vi "motion_generate_test_withvelocitycontrol_withswingdelay_motor4.vi"() -> ()   [LabVIEW 2017]
uses:
  Downloads/Interfacing File 1/Software_Driver/DynamixelSDK/DynamixelSDK-master/labview/dxl_x86_c.lvlib/dxl_x86_c.lvlib
panel:
  in  "ADDR_MX_GOAL_Velocity 2":u8=5
  in  "data 3":u16
  in  "data 2":u16
  in  "data":u16
  in  "ADDR_MX_GOAL_Velocity":u8=5
  in  "angle 2":dbl=180.0
  in  "motor3 2":dbl=220.0
  in  "motor1&2 2":dbl=150.0
  in  "z축 선택":dbl
  in  "motor1&2":dbl=150.0
  in  "motor3":dbl=220.0
  in  "angle":dbl=180.0
  in  "Boolean":bool
  in  "positioning time_2":u32
  in  "positioning time_1":u32
  in  "initial_5":dbl=230.0
  in  "initial_4":dbl=180.0
  out "value : MX (knob)\npresent position 4":u16(knob)
  in  "dynamixel_id 4":u8=4
  out "protocol_version 2":dbl=2.0
  in  "ADDR_MX_\nPRESENT_POSITION 2":u16=132
  out "dynamixel_error 2":string
  out "dynamixel_comm_result  2":string
  in  "ADDR_MX_\nGOAL_POSITION 2":u16=116
  in  "ADDR_MX_\nTORQUE_ENABLE 2":u16=64
  in  "initial_3":dbl=260.0
  in  "initial_1&2":dbl=230.0
  out "value : MX (knob)\npresent position 3":u16(knob)
  out "value : MX (knob)\npresent position 2":u16(knob)
  out "value : MX (knob)\npresent position":u16(knob)
  in  "dynamixel_id 3":u8=3
  in  "dynamixel_id 2":u8=2
  out "dynamixel_comm_result":string
  out "dynamixel_error":string
  in  "device_name":string="COM3"
  in  "ADDR_MX_\nPRESENT_POSITION":u16=36
  in  "ADDR_MX_\nGOAL_POSITION":u16=30
  in  "ADDR_MX_\nTORQUE_ENABLE":u16=24
  out "protocol_version":dbl=1.0
  in  "terminate":bool
  out "port_num":i32
  in  "dynamixel_id":u8=1
  in  "baud_rate":i32=57600
  # "Motor connection status"
  # "Time set"
  # "Sensing data"
  # "Handler setup"
  # "link length"
  # "initial angle"
  # "desired angle"
  # "*각 관절에 모터 연결 시 180도 라인 기준으로 연결 시키기 \n(-각도 반영해주기 위함!) \n-> 모터 input은 -180~180까지 계산됨!"
  # "*yaw motor는 0도 라인 기준으로 연결 시키기"
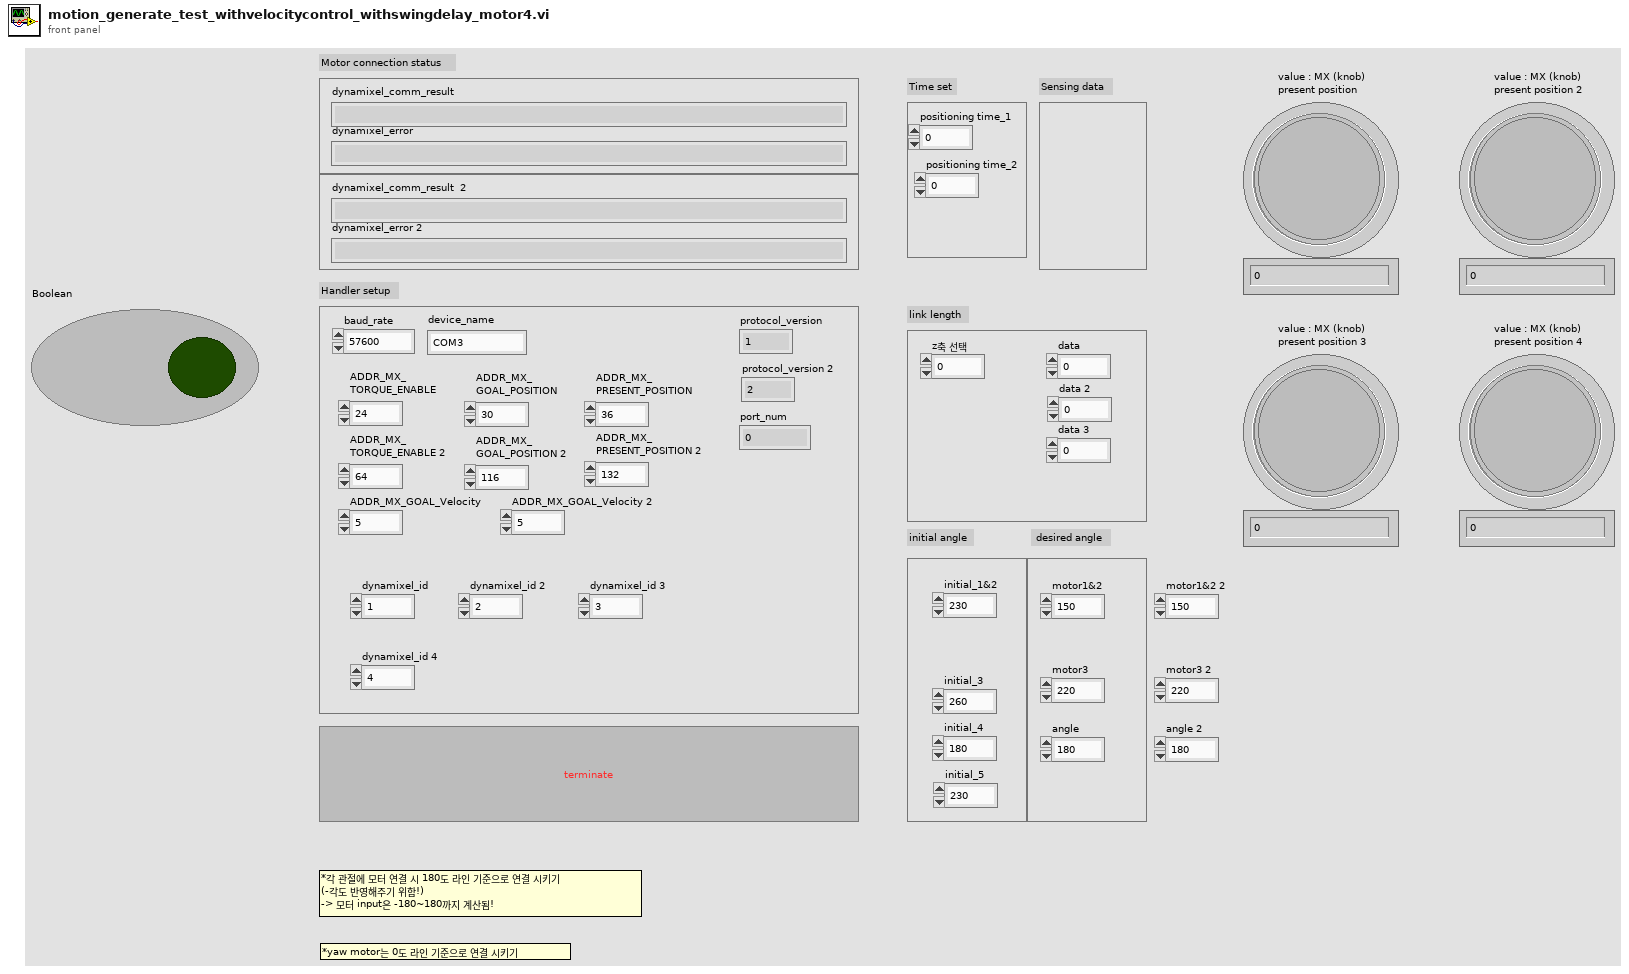
[diagram p1: front panel]
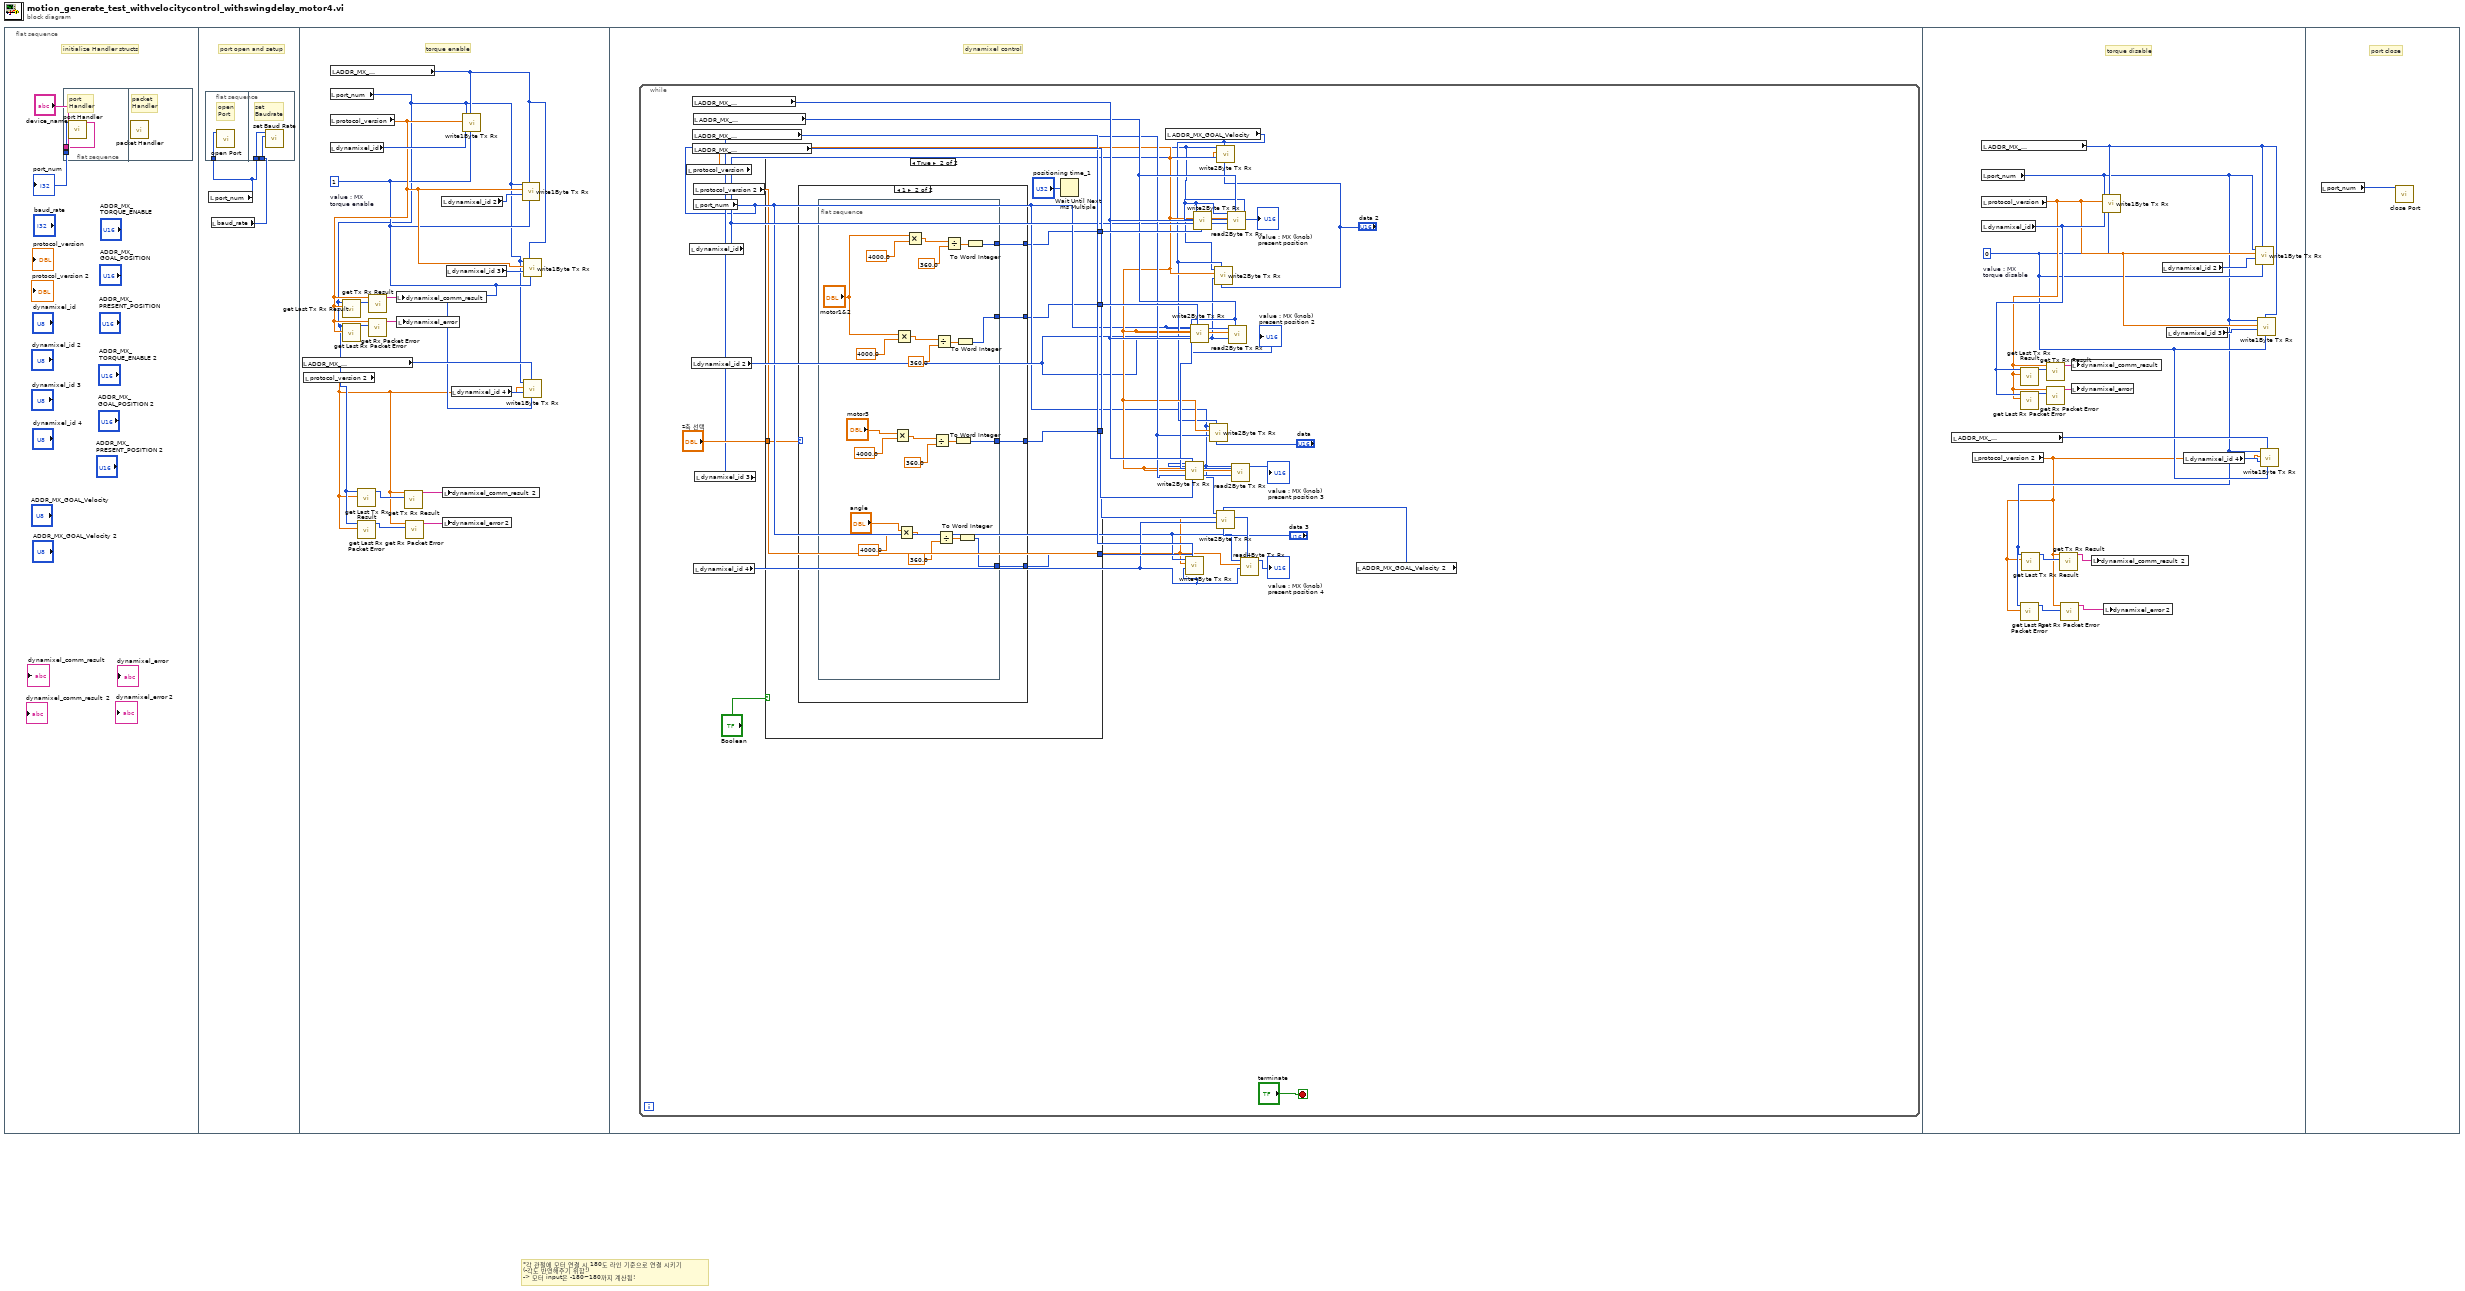
[diagram p0: block diagram]
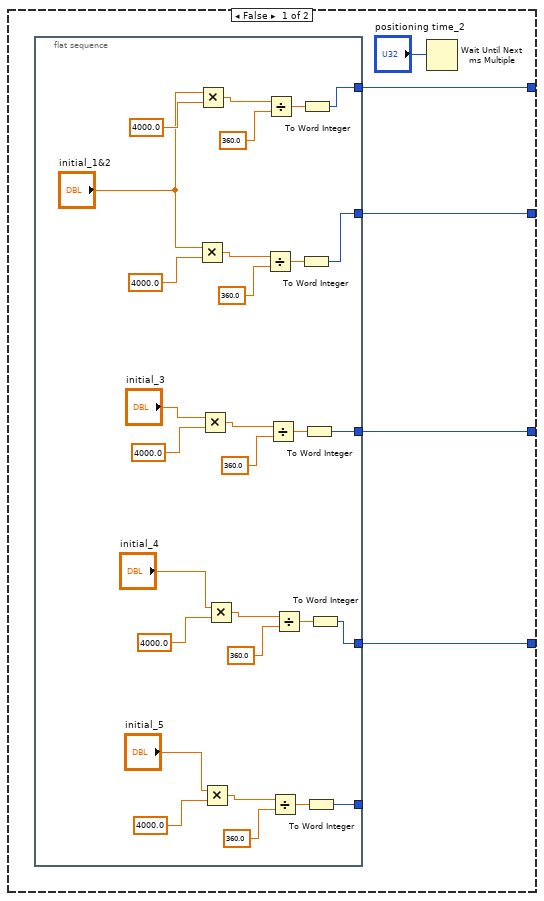
[diagram p2: hidden frame]
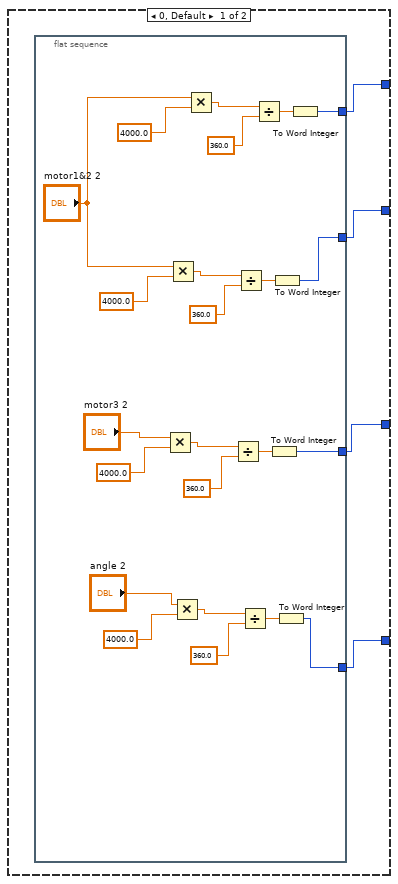
[diagram p3: hidden frame]
diagram:
  # "*각 관절에 모터 연결 시 180도 라인 기준으로 연결 시키기 \n(-각도 반영해주기 위함!) \n-> 모터 input은 -180~180까지 계산됨!"
  n1 = flat-sequence {
    frame #0 {
      # "initialize Handler structs"
      n2 = flat-sequence {
        tunnel: [w4] -> w2
        tunnel: "device_name" -> [w3]
        frame #0 {
          # "port\nHandler"
          n3 = call "port Handler.vi"("port_name"=w3) -> ("function return"=w4:i32)  [unwired: 10 in]
        }
        frame #1 {
          # "packet\nHandler"
          n4 = call "packet Handler.vi"() -> ()  [unwired: 12 in]
        }
      }
      "port_num" <- w2
    }
    frame #1 {
      # "port open and setup"
      n5 = flat-sequence {
        tunnel: w6 -> [w7]
        tunnel: w6 -> [w9]
        tunnel: w5 -> [w8]
        frame #0 {
          # "open\nPort"
          n6 = call "open Port.vi"("port_num"=w7) -> ()  [unwired: 10 in, 1 out]
        }
        frame #1 {
          # "set\nBaudrate"
          n7 = call "set Baud Rate.vi"("baudrate"=w8, "port_num"=w9) -> ()  [unwired: 9 in, 1 out]
        }
      }
      n8 = local read "port_num"() -> (w6:i32)
      n9 = local read "baud_rate"() -> (w5:i32)
    }
    frame #2 {
      w16 = 1  # value : MX torque enable
      # "torque enable"
      n10 = local read "ADDR_MX_\nTORQUE_ENABLE 2"() -> (w17:u16)
      n11 = local read "protocol_version 2"() -> (w10:dbl)
      n12 = local read "port_num"() -> (w11:i32)
      n13 = local read "protocol_version"() -> (w20:dbl)
      n14 = local read "dynamixel_id"() -> (w27:u8)
      n15 = local read "ADDR_MX_\nTORQUE_ENABLE"() -> (w19:u16)
      n16 = call "get Last Tx Rx Result.vi"("protocol_version"=w20, "port_num"=w11) -> ("function return"=w23:i32)  [unwired: 9 in]
      n17 = call "get Last Rx Packet Error.vi"("protocol_version"=w20, "port_num"=w11) -> ("function return"=w24:u8)  [unwired: 9 in]
      n18 = call "get Last Rx Packet Error.vi"("protocol_version"=w10, "port_num"=w11) -> ("function return"=w13:u8)  [unwired: 9 in]
      n19 = call "get Last Tx Rx Result.vi"("protocol_version"=w10, "port_num"=w11) -> ("function return"=w15:i32)  [unwired: 9 in]
      n20 = call "get Rx Packet Error.vi"("error"=w24, "protocol_version"=w20) -> ("function return"=w26:string)  [unwired: 9 in]
      n21 = call "get Tx Rx Result.vi"("result"=w23, "protocol_version"=w20) -> ("function return"=w25:string)  [unwired: 9 in]
      n22 = local write "dynamixel_comm_result"(w25) -> ()
      n23 = local write "dynamixel_error"(w26) -> ()
      n24 = call "get Tx Rx Result.vi"("result"=w15, "protocol_version"=w10) -> ("function return"=w14:string)  [unwired: 9 in]
      n25 = call "get Rx Packet Error.vi"("error"=w13, "protocol_version"=w10) -> ("function return"=w12:string)  [unwired: 9 in]
      n26 = local read "dynamixel_id 2"() -> (w22:u8)
      n27 = local write "dynamixel_comm_result  2"(w14) -> ()
      n28 = local write "dynamixel_error 2"(w12) -> ()
      n29 = local read "dynamixel_id 3"() -> (w21:u8)
      n30 = local read "dynamixel_id 4"() -> (w18:u8)
      n31 = call "write1Byte Tx Rx.vi"("data"=w16, "address"=w19, "id"=w27, "protocol_version"=w20, "port_num"=w11) -> ()  [unwired: 7 in]
      n32 = call "write1Byte Tx Rx.vi"("data"=w16, "address"=w19, "id"=w22, "protocol_version"=w20, "port_num"=w11) -> ()  [unwired: 7 in]
      n33 = call "write1Byte Tx Rx.vi"("data"=w16, "address"=w19, "id"=w21, "protocol_version"=w20, "port_num"=w11) -> ()  [unwired: 7 in]
      n34 = call "write1Byte Tx Rx.vi"("data"=w16, "address"=w17, "id"=w18, "protocol_version"=w10, "port_num"=w11) -> ()  [unwired: 7 in]
    }
    frame #3 {
      # "dynamixel control"
      n35 = while {
        stop <- "terminate" stop-if-true
        n36 = local read "protocol_version"() -> (w36:dbl)
        n37 = local read "dynamixel_id"() -> (w37:u8)
        n38 = local read "dynamixel_id 2"() -> (w35:u8)
        n39 = local read "ADDR_MX_\nGOAL_POSITION"() -> (w51:u16)
        n40 = local read "ADDR_MX_\nGOAL_POSITION 2"() -> (w43:u16)
        n41 = local read "ADDR_MX_\nPRESENT_POSITION 2"() -> (w44:u16)
        n42 = local read "ADDR_MX_\nPRESENT_POSITION"() -> (w50:u16)
        n43 = local read "protocol_version 2"() -> (w29:dbl)
        n44 = local read "port_num"() -> (w30:i32)
        n45 = local read "dynamixel_id 4"() -> (w33:u8)
        n46 = local read "dynamixel_id 3"() -> (w39:u8)
        n47 = case shown="True" "Boolean" {
          tunnel: [w59 w94] -> w53
          tunnel: [w58 w93] -> w52
          tunnel: [w57 w92] -> w49
          tunnel: [w56 w91] -> w42
          tunnel: "z축 선택" -> [_ w89]
          frame False {
            n48 = flat-sequence {
              tunnel: [w84] -> w59
              tunnel: [w74] -> w58
              tunnel: [w73] -> w57
              tunnel: [w64] -> w56
              tunnel: [w63] -> _
              frame #0 {
                n49 = Multiply(x="initial_1&2", y=4000.0) -> (x*y=w82:dbl)
                n50 = Multiply(x="initial_1&2", y=4000.0) -> (x*y=w87:dbl)
                n51 = Multiply(x="initial_3", y=4000.0) -> (x*y=w78:dbl)
                n52 = Multiply(x="initial_5", y=4000.0) -> (x*y=w67:dbl)
                n53 = Multiply(x="initial_4", y=4000.0) -> (x*y=w71:dbl)
                n54 = Divide(x=w82, y=360.0) -> (x/y=w80:dbl)
                n55 = Divide(x=w87, y=360.0) -> (x/y=w85:dbl)
                n56 = Divide(x=w78, y=360.0) -> (x/y=w76:dbl)
                n57 = Divide(x=w67, y=360.0) -> (x/y=w65:dbl)
                n58 = Divide(x=w71, y=360.0) -> (x/y=w69:dbl)
                n59 = To Word Integer(number=w80) -> (16bit integer=w74:i16)
                n60 = To Word Integer(number=w85) -> (16bit integer=w84:i16)
                n61 = To Word Integer(number=w76) -> (16bit integer=w73:i16)
                n62 = To Word Integer(number=w65) -> (16bit integer=w63:i16)
                n63 = To Word Integer(number=w69) -> (16bit integer=w64:i16)
              }
            }
            n64 = Wait Until Next ms Multiple(millisecond multiple="positioning time_2") -> ()  [unwired: 1 out]
          }
          frame True {
            n65 = case shown="1" w89 {
              tunnel: [w95 w125] -> w94
              tunnel: [w96 w124] -> w93
              tunnel: [w97 w123] -> w92
              tunnel: [w98 w122] -> w91
              frame 0, Default {
                n66 = flat-sequence {
                  tunnel: [w117] -> w95
                  tunnel: [w112] -> w96
                  tunnel: [w103] -> w98
                  tunnel: [w99] -> w97
                  frame #0 {
                    n67 = Multiply(x="motor3 2", y=4000.0) -> (x*y=w110:dbl)
                    n68 = Multiply(x="motor1&2 2", y=4000.0) -> (x*y=w115:dbl)
                    n69 = Multiply(x="angle 2", y=4000.0) -> (x*y=w106:dbl)
                    n70 = Multiply(x="motor1&2 2", y=4000.0) -> (x*y=w120:dbl)
                    n71 = Divide(x=w110, y=360.0) -> (x/y=w108:dbl)
                    n72 = Divide(x=w115, y=360.0) -> (x/y=w113:dbl)
                    n73 = Divide(x=w106, y=360.0) -> (x/y=w104:dbl)
                    n74 = Divide(x=w120, y=360.0) -> (x/y=w118:dbl)
                    n75 = To Word Integer(number=w108) -> (16bit integer=w99:i16)
                    n76 = To Word Integer(number=w113) -> (16bit integer=w112:i16)
                    n77 = To Word Integer(number=w104) -> (16bit integer=w103:i16)
                    n78 = To Word Integer(number=w118) -> (16bit integer=w117:i16)
                  }
                }
              }
              frame 1 {
                n79 = flat-sequence {
                  tunnel: [w144] -> w125
                  tunnel: [w139] -> w124
                  tunnel: [w134] -> w123
                  tunnel: [w129] -> w122
                  frame #0 {
                    n80 = Multiply(x="motor3", y=4000.0) -> (x*y=w137:dbl)
                    n81 = Multiply(x="motor1&2", y=4000.0) -> (x*y=w142:dbl)
                    n82 = Multiply(x="angle", y=4000.0) -> (x*y=w132:dbl)
                    n83 = Multiply(x="motor1&2", y=4000.0) -> (x*y=w147:dbl)
                    n84 = Divide(x=w137, y=360.0) -> (x/y=w135:dbl)
                    n85 = Divide(x=w142, y=360.0) -> (x/y=w140:dbl)
                    n86 = Divide(x=w132, y=360.0) -> (x/y=w130:dbl)
                    n87 = Divide(x=w147, y=360.0) -> (x/y=w145:dbl)
                    n88 = To Word Integer(number=w135) -> (16bit integer=w134:i16)
                    n89 = To Word Integer(number=w140) -> (16bit integer=w139:i16)
                    n90 = To Word Integer(number=w130) -> (16bit integer=w129:i16)
                    n91 = To Word Integer(number=w145) -> (16bit integer=w144:i16)
                  }
                }
              }
            }
            n92 = Wait Until Next ms Multiple(millisecond multiple="positioning time_1") -> ()  [unwired: 1 out]
          }
        }
        n93 = local read "ADDR_MX_GOAL_Velocity"() -> (w31:u8)
        n94 = call "write2Byte Tx Rx.vi"("data"=w49, "address"=w51, "id"=w39, "protocol_version"=w36, "port_num"=w30) -> ()  [unwired: 7 in]
        n95 = call "write4Byte Tx Rx.vi"("data"=w42, "address"=w43, "id"=w33, "protocol_version"=w29, "port_num"=w30) -> ()  [unwired: 7 in]
        n96 = call "write2Byte Tx Rx.vi"("data"=w52, "address"=w51, "id"=w35, "protocol_version"=w36, "port_num"=w30) -> ()  [unwired: 7 in]
        n97 = call "write2Byte Tx Rx.vi"("data"=w53, "address"=w51, "id"=w37, "protocol_version"=w36, "port_num"=w30) -> ()  [unwired: 7 in]
        n98 = call "write2Byte Tx Rx.vi"("data"="data", "address"=w31, "id"=w39, "protocol_version"=w36, "port_num"=w30) -> ()  [unwired: 7 in]
        n99 = call "write2Byte Tx Rx.vi"("data"="data 2", "address"=w31, "id"=w35, "protocol_version"=w36, "port_num"=w30) -> ()  [unwired: 7 in]
        n100 = call "write2Byte Tx Rx.vi"("data"="data 2", "address"=w31, "id"=w37, "protocol_version"=w36, "port_num"=w30) -> ()  [unwired: 7 in]
        n101 = call "read2Byte Tx Rx.vi"("address"=w50, "id"=w37, "protocol_version"=w36, "port_num"=w30) -> ("function return"=→"value : MX (knob)\npresent position":u16)  [unwired: 7 in]
        n102 = call "read2Byte Tx Rx.vi"("address"=w50, "id"=w35, "protocol_version"=w36, "port_num"=w30) -> ("function return"=→"value : MX (knob)\npresent position 2":u16)  [unwired: 7 in]
        n103 = call "read2Byte Tx Rx.vi"("address"=w50, "id"=w39, "protocol_version"=w36, "port_num"=w30) -> ("function return"=→"value : MX (knob)\npresent position 3":u16)  [unwired: 7 in]
        n104 = call "read4Byte Tx Rx.vi"("address"=w44, "id"=w33, "protocol_version"=w29, "port_num"=w30) -> ("function return"=→"value : MX (knob)\npresent position 4":u32)  [unwired: 7 in]
        n105 = local read "ADDR_MX_GOAL_Velocity 2"() -> (w28:u8)
        n106 = call "write2Byte Tx Rx.vi"("data"="data 3", "address"=w28, "id"=w33, "protocol_version"=w29, "port_num"=w30) -> ()  [unwired: 7 in]
      }
    }
    frame #4 {
      w155 = 0  # value : MX torque disable
      # "torque disable"
      n107 = local read "ADDR_MX_\nTORQUE_ENABLE 2"() -> (w156:u16)
      n108 = local read "protocol_version 2"() -> (w151:dbl)
      n109 = local read "port_num"() -> (w153:i32)
      n110 = local read "ADDR_MX_\nTORQUE_ENABLE"() -> (w158:u16)
      n111 = local read "protocol_version"() -> (w159:dbl)
      n112 = local read "dynamixel_id"() -> (w162:u8)
      n113 = call "get Last Rx Packet Error.vi"("protocol_version"=w151, "port_num"=w153) -> ("function return"=w152:u8)  [unwired: 9 in]
      n114 = call "get Last Tx Rx Result.vi"("protocol_version"=w159, "port_num"=w162) -> ("function return"=w164:i32)  [unwired: 9 in]
      n115 = call "get Last Rx Packet Error.vi"("protocol_version"=w159, "port_num"=w162) -> ("function return"=w163:u8)  [unwired: 9 in]
      n116 = call "get Last Tx Rx Result.vi"("protocol_version"=w151, "port_num"=w153) -> ("function return"=w154:i32)  [unwired: 9 in]
      n117 = call "get Tx Rx Result.vi"("result"=w164, "protocol_version"=w159) -> ("function return"=w165:string)  [unwired: 9 in]
      n118 = call "get Rx Packet Error.vi"("error"=w163, "protocol_version"=w159) -> ("function return"=w166:string)  [unwired: 9 in]
      n119 = call "get Tx Rx Result.vi"("result"=w154, "protocol_version"=w151) -> ("function return"=w149:string)  [unwired: 9 in]
      n120 = call "get Rx Packet Error.vi"("error"=w152, "protocol_version"=w151) -> ("function return"=w150:string)  [unwired: 9 in]
      n121 = local write "dynamixel_comm_result"(w165) -> ()
      n122 = local write "dynamixel_error"(w166) -> ()
      n123 = local write "dynamixel_comm_result  2"(w149) -> ()
      n124 = call "write1Byte Tx Rx.vi"("data"=w155, "address"=w158, "id"=w162, "protocol_version"=w159, "port_num"=w153) -> ()  [unwired: 7 in]
      n125 = local write "dynamixel_error 2"(w150) -> ()
      n126 = local read "dynamixel_id 2"() -> (w161:u8)
      n127 = local read "dynamixel_id 3"() -> (w160:u8)
      n128 = local read "dynamixel_id 4"() -> (w157:u8)
      n129 = call "write1Byte Tx Rx.vi"("data"=w155, "address"=w158, "id"=w161, "protocol_version"=w159, "port_num"=w153) -> ()  [unwired: 7 in]
      n130 = call "write1Byte Tx Rx.vi"("data"=w155, "address"=w158, "id"=w160, "protocol_version"=w159, "port_num"=w153) -> ()  [unwired: 7 in]
      n131 = call "write1Byte Tx Rx.vi"("data"=w155, "address"=w156, "id"=w157, "protocol_version"=w151, "port_num"=w153) -> ()  [unwired: 7 in]
    }
    frame #5 {
      # "port close"
      n132 = local read "port_num"() -> (w167:i32)
      n133 = call "close Port.vi"("port_num"=w167) -> ()  [unwired: 11 in]
    }
  }
